vi "SID4 GEECS save measurement.vi"(7 "PHASE":sgl[][](array[numeric]), 8 "error in (no error)":errorcluster, 9 "INTENSITY":sgl[][](array[numeric]), 10 "Interferogram path":path, 11 "Refnum in":T1) -> (0 "error out":errorcluster, 2 "Saved Phase file":path, 3 "Intensity file":path)   [LabVIEW 2013]
uses:
  Program Files (x86)/SID4_SDK/SDKSID4_Types.llb/Refnum SDKSID4 session.ctl
  <userlib>/_OpenG.lib/file/file.llb/File Exists - Scalar__ogtk.vi
  <userlib>/_OpenG.lib/file/file.llb/Strip Path Extension - Path__ogtk.vi
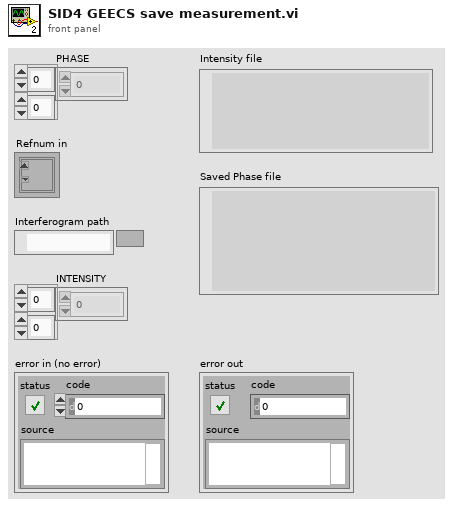
[diagram p1: front panel]
types:
  T1 = typedef "Refnum SDKSID4 session.ctl" = refnum<k1>
  T2 = typedef "Image Type" = u32
  T3 = typedef "IMAQ Image.ctl" = refnum<image>
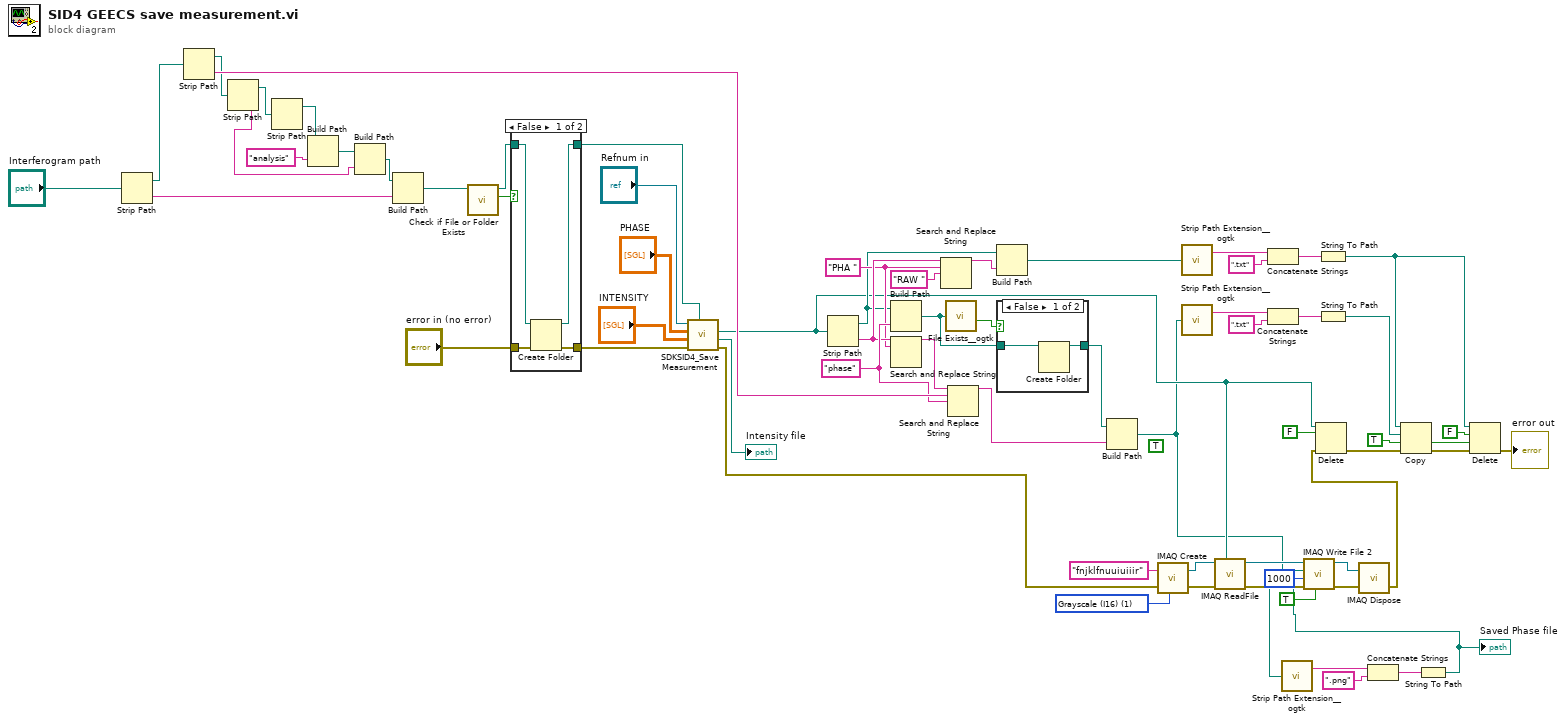
[diagram p0: block diagram]
diagram:
  w17 = T2 1 items=["Grayscale (U8)", "Grayscale (I16)", "Grayscale (SGL)", "Complex (CSG)", "RGB (U32)", "HSL (U32)", "RGB (U64)", "Grayscale (U16)"] ("Image Type")
  (unwired) TRUE ("overwrite (F)")
  w50 = "phase" ("replace string (\"\")")
  w43 = "PHA " ("search string")
  n1 = Strip Path(path="Interferogram path") -> (stripped path=w52:path, name=w63:string)
  n2 = Strip Path(path=w52) -> (stripped path=w24:path, name=w51:string)
  n3 = Strip Path(path=w24) -> (stripped path=w23:path, name=w19:string)
  n4 = Strip Path(path=w23) -> (stripped path=w22:path)  [unwired: 1 out]
  n5 = Build Path(base path=w22, name or relative path="analysis") -> (appended path=w21:path)
  n6 = Build Path(base path=w21, name or relative path=w19) -> (appended path=w20:path)
  n7 = Build Path(base path=w20, name or relative path=w63) -> (appended path=w64:path)
  n8 = call <vilib>:"Check if File or Folder Exists.vi"("path"=w64) -> ("file or folder exists?"=w58:bool, "dup path"=w59:path)  [unwired: 8 in, 1 out]
  n9 = case shown="False" w58 {
    tunnel: w59 -> [w70 w72]
    tunnel: [w69 w72] -> w60
    tunnel: "error in (no error)" -> [w68 w71]
    tunnel: [w67 w71] -> w62
    frame False {
      n10 = Create Folder(path (use dialog)=w70, error in=w68) -> (created path=w69:path, error out=w67:errorcluster)  [unwired: 1 in, 1 out]
    }
    frame True {
    }
  }
  n11 = call "SDKSID4_Save Measurement.vi"("Generic path"=w60, "error in (no error)"=w62, "Intensity"="INTENSITY", "Phase"="PHASE", "SDKSID4 session In"="Refnum in") -> ("error out"=w13:errorcluster, "Intensity file"=→"Intensity file":path, "Phase file"=w16:path)  [unwired: 1 out]
  n12 = Strip Path(path=w16) -> (stripped path=w41:path, name=w44:string)
  n13 = Build Path(base path=w41, name or relative path=w50) -> (appended path=w48:path)
  n14 = Search and Replace String(input string=w44, search string=w43) -> (result string=w53:string)  [unwired: 6 in, 3 out]
  n15 = Search and Replace String(input string=w44, search string=w43, replace string="RAW " ("search string")) -> (result string=w40:string)  [unwired: 5 in, 3 out]
  n16 = call-poly <userlib>:"File Exists__ogtk.vi"("file path"=w48) -> ("exists"=w49:bool)  [unwired: 6 in, 1 out]
  n17 = Search and Replace String(input string=w53, search string=w51, replace string=w50) -> (result string=w46:string)  [unwired: 5 in, 3 out]
  n18 = Build Path(base path=w41, name or relative path=w40) -> (appended path=w26:path)
  n19 = case shown="False" w49 {
    tunnel: [w73 w75] -> w47
    tunnel: w48 -> [w74 w75]
    frame False {
      n20 = Create Folder(path (use dialog)=w74) -> (created path=w73:path)  [unwired: 2 in, 2 out]
    }
    frame True {
    }
  }
  n21 = Build Path(base path=w47, name or relative path=w46) -> (appended path=w4:path)
  n22 = call "IMAQ Create"("Image Name"="fnjklfnuuiuiiir", "Image Type"=w17, "error in (no error)"=w13) -> ("New Image"=w15:T3, "error out"=w12:errorcluster)  [unwired: 2 in]
  n23 = call-poly <userlib>:"Strip Path Extension__ogtk.vi"("path"=w26) -> ("root"=w27:string)  [unwired: 1 out]
  n24 = call-poly <userlib>:"Strip Path Extension__ogtk.vi"("path"=w4) -> ("root"=w33:string)  [unwired: 1 out]
  n25 = call "IMAQ ReadFile"("File Path"=w16, "error in (no error)"=w12, "Image"=w15) -> ("error out"=w11:errorcluster, "Image Out"=w14:T3)  [unwired: 4 in, 3 out]
  n26 = Concatenate Strings(w27, ".txt" ("string")) -> (w29:string)
  n27 = Concatenate Strings(w33, ".txt" ("string")) -> (w31:string)
  n28 = call-poly <userlib>:"Strip Path Extension__ogtk.vi"("path"=w4) -> ("root"=w5:string)  [unwired: 1 out]
  n29 = String To Path(string=w29) -> (path=w25:path)
  n30 = String To Path(string=w31) -> (path=w30:path)
  n31 = Concatenate Strings(w5, ".png" ("string")) -> (w7:string)
  n32 = String To Path(string=w7) -> (path=w3:path)
  "Saved Phase file" <- w3
  n33 = call-poly "IMAQ Write File 2"("Use bit depth? (false)"=TRUE, "error in (no error)"=w11, "Image Quality"=u32 1000, "File Path"=w3, "Image"=w14) -> ("error out"=w9:errorcluster, "Image Out (duplicate)"=w10:T3)  [unwired: 5 in]
  n34 = call "IMAQ Dispose"("Image"=w10, "error in (no error)"=w9) -> ("error out"=w8:errorcluster)  [unwired: 4 in]
  n35 = Delete(path (use dialog)=w16, entire hierarchy (F)=FALSE, error in=w8) -> (error out=w35:errorcluster)  [unwired: 2 in, 2 out]
  n36 = Copy(8:w35, 9:TRUE ("overwrite (F)"), 10:w30, 11:w25) -> (0:w37:errorcluster, 1:w38:bool)  [unwired: 1 in, 1 out]
  n37 = Delete(path (use dialog)=w25, entire hierarchy (F)=FALSE, confirm (F)=w38, error in=w37) -> (error out=→"error out":errorcluster)  [unwired: 1 in, 2 out]
